vi "UT_LogRecord_Main.vi"(8 "error in":errorcluster) -> (0 "error out":errorcluster)   [LabVIEW 2016, in "UT_LogRecord.lvlib"]
doc: "Collection of tests for the LogRecord class."
uses:
  UT_LogRecord.lvlib
  <vilib>/addons/_JKI Toolkits/Caraya/classes/Test/Test.lvclass
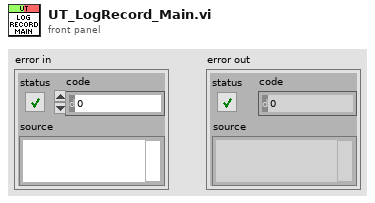
[diagram p1: front panel]
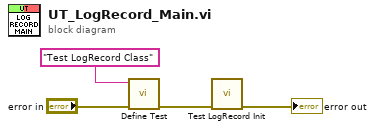
[diagram p0: block diagram]
diagram:
  n1 = call <vilib>:"Define Test.vi"("error in (no error)"="error in", "Label (VI Title)"="Test LogRecord Class") -> ("error out"=w3:errorcluster)  [unwired: 8 in, 1 out]
  n2 = call "Test LogRecord Init.vi"("error in"=w3) -> ("error out"=→"error out":errorcluster)  [unwired: 10 in]
